vi "convertData.vi"(8 "error in (no error)":errorcluster, 10 "continuous":bool=TRUE, 11 "SpinCore in":refnum<class "SpinCore.lvclass">) -> (0 "error out":errorcluster, 2 "Instructions":T1(array[cluster]) {"Op Code" items=["Continue", "Stop", "Loop", "End Loop", "JSR", "RTS", "Branch", "Long Delay", "Wait"]; "Amp Register2" items=["0", "1", "2", "3"]; "Phase Register2" items=["0", "1", "2", "3", "4", "5", "6", "7", "8", "9", "10", "11", "12", "13", "14", "15"]; "Freq Register2" items=["0", "1", "2", "3", "4", "5", "6", "7", "8", "9", "10", "11", "12", "13", "14", "15"]; "Amp Register1" items=["0", "1", "2", "3"]; "Phase Register1" items=["0", "1", "2", "3", "4", "5", "6", "7", "8", "9", "10", "11", "12", "13", "14", "15"]; "Freq Register1" items=["0", "1", "2", "3", "4", "5", "6", "7", "8", "9", "10", "11", "12", "13", "14", "15"]; "Length" format="%.3p"}, 3 "SpinCore out":refnum<class "SpinCore.lvclass">)   [LabVIEW 2009, in "Hardware.lvlib" / "Channels.lvlib" / "SpinCore.lvclass"]
uses:
  SpinCore.lvclass
  SpinCore.lvclass/SpinCore.ctl
panel:
  # "0"
  # "1"
  # "2"
  # "3"
  # "4"
  # "5"
  # "6"
  # "7"
  # "8"
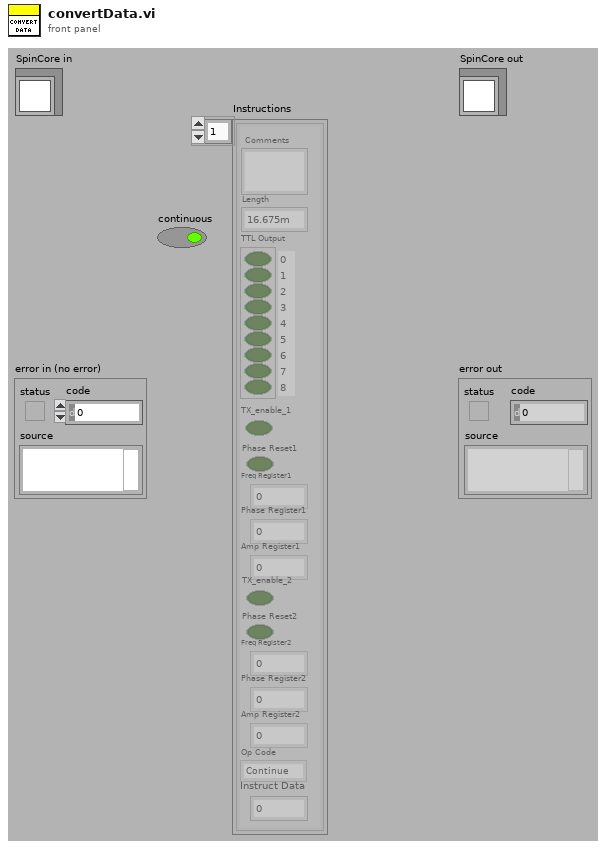
[diagram p1: front panel]
types:
  T1 = cluster{"Comments":string, "Length":dbl, "TTL Output":bool[], "TX_enable_1":bool, "Phase Reset1":bool, "Freq Register1":i32, "Phase Register1":i32, "Amp Register1":i32, "TX_enable_2":bool, "Phase Reset2":bool, "Freq Register2":i32, "Phase Register2":i32, "Amp Register2":i32, "Instruct Data":i32, "Op Code":i32}[]
  T2 = cluster{"Comments":string, "Length":dbl, "TTL Output":bool[], "TX_enable_0":bool, "Phase Reset0":bool, "Freq Register0":i32, "Phase Register0":i32, "Amp Register0":i32, "TX_enable_1":bool, "Phase Reset1":bool, "Freq Register1":i32, "Phase Register1":i32, "Amp Register1":i32, "Instruct Data":i32, "Op Code":i32}[]
  T3 = cluster{"Comments":string, "Length":dbl, "TTL Output":bool[], "TX_enable_1":bool, "Phase Reset1":bool, "Freq Register1":i32, "Phase Register1":i32, "Amp Register1":i32, "TX_enable_2":bool, "Phase Reset2":bool, "Freq Register2":i32, "Phase Register2":i32, "Amp Register2":i32, "Instruct Data":i32, "Op Code":i32}
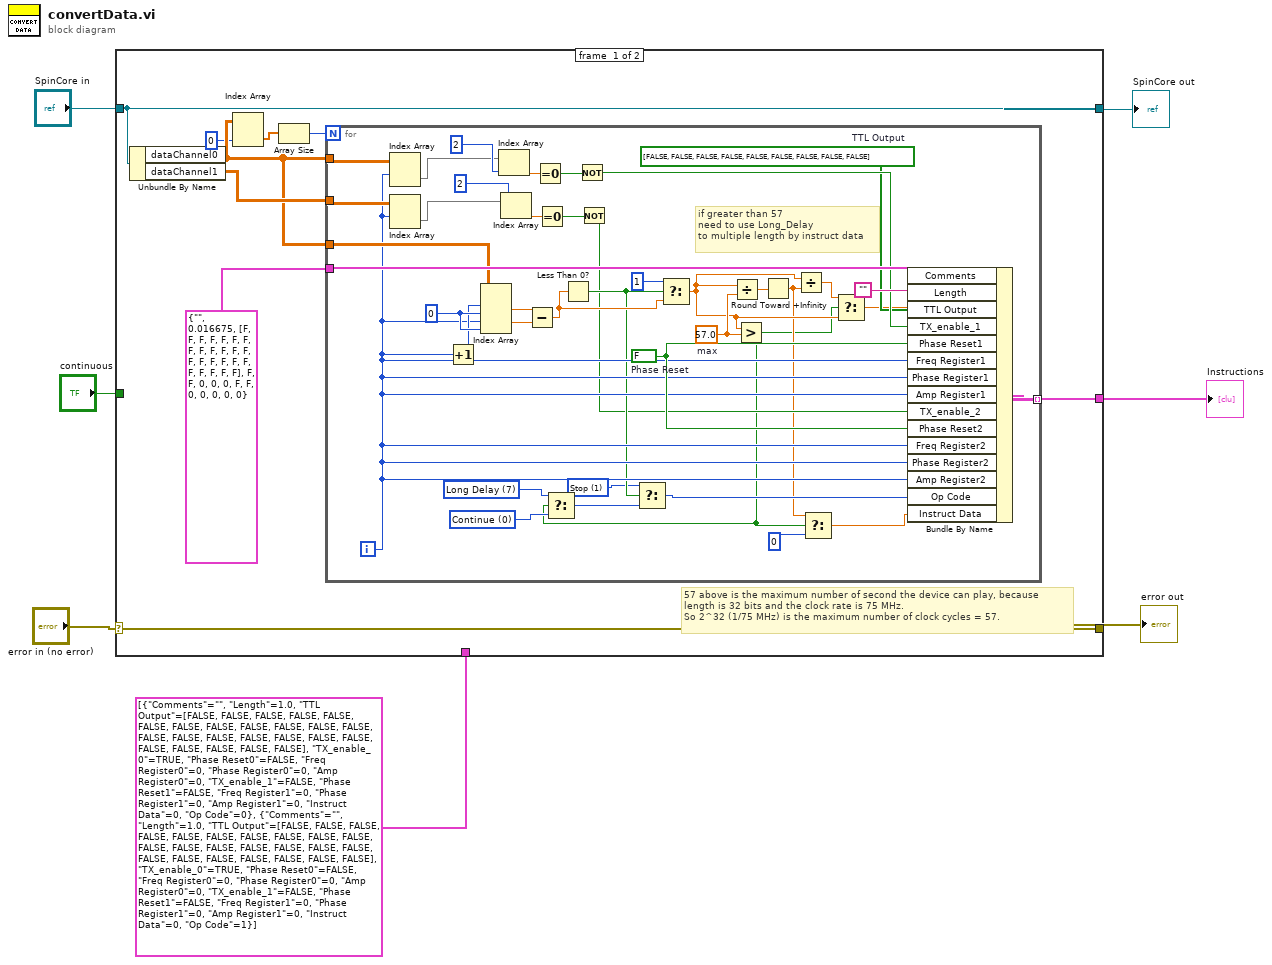
[diagram p0: block diagram]
diagram:
  n1 = case shown="No Error" "error in (no error)" {
    selector: "error in (no error)" -> [w16 w58]
    tunnel: [w16 w58] -> w6
    tunnel: [w15 w57] -> w4
    tunnel: "SpinCore in" -> [w15 w57]
    tunnel: [w8 _] -> w3
    tunnel: T2 [{"Comments"="", "Length"=1.0, "TTL Output"=[FALSE, FALSE, FALSE, FALSE, FALSE, FALSE, FALSE, FALSE, FALSE, FALSE, FALSE, FALSE, FALSE, FALSE, FALSE, FALSE, FALSE, FALSE, FALSE, FALSE, FALSE, FALSE, FALSE, FALSE], "TX_enable_0"=TRUE, "Phase Reset0"=FALSE, "Freq Register0"=0, "Phase Register0"=0, "Amp Register0"=0, "TX_enable_1"=FALSE, "Phase Reset1"=FALSE, "Freq Register1"=0, "Phase Register1"=0, "Amp Register1"=0, "Instruct Data"=0, "Op Code"=0}, {"Comments"="", "Length"=1.0, "TTL Output"=[FALSE, FALSE, FALSE, FALSE, FALSE, FALSE, FALSE, FALSE, FALSE, FALSE, FALSE, FALSE, FALSE, FALSE, FALSE, FALSE, FALSE, FALSE, FALSE, FALSE, FALSE, FALSE, FALSE, FALSE], "TX_enable_0"=TRUE, "Phase Reset0"=FALSE, "Freq Register0"=0, "Phase Register0"=0, "Amp Register0"=0, "TX_enable_1"=FALSE, "Phase Reset1"=FALSE, "Freq Register1"=0, "Phase Register1"=0, "Amp Register1"=0, "Instruct Data"=0, "Op Code"=1}] ("Instructions") -> [_ _]
    tunnel: "continuous" -> [_ _]
    frame #0 {
      # "57 above is the maximum number of second the device can play, because\nlength is 32 bits and the clock rate is 75 MHz.\nSo 2^32 (1/75 MHz) is the maximum number of clock cycles = 57."
      n2 = Unbundle By Name(w15) -> ("dataChannel0"=w13:dbl[][], "dataChannel1"=w14:dbl[][])
      n3 = Index Array(array=w13, index (col)=0) -> (element=w12:dbl[])  [unwired: 1 in]
      n4 = Array Size(array=w12) -> (size(s)=w10:i32)
      n5 = for {
        N: w10 -> [_]
        tunnel: w13 -> [w39]
        tunnel: w14 -> [w37]
        tunnel: T3 {"Comments"="", "Length"=0.016675, "TTL Output"=[FALSE, FALSE, FALSE, FALSE, FALSE, FALSE, FALSE, FALSE, FALSE, FALSE, FALSE, FALSE, FALSE, FALSE, FALSE, FALSE, FALSE, FALSE, FALSE, FALSE, FALSE, FALSE, FALSE, FALSE], "TX_enable_1"=FALSE, "Phase Reset1"=FALSE, "Freq Register1"=0, "Phase Register1"=0, "Amp Register1"=0, "TX_enable_2"=FALSE, "Phase Reset2"=FALSE, "Freq Register2"=0, "Phase Register2"=0, "Amp Register2"=0, "Instruct Data"=0, "Op Code"=0} ("DDS-II Instruction") -> [w50]
        tunnel: w13 -> [w48]
        tunnel: [w43] -> w8 mode=indexing
        i -> [w36]
        w23 = 57.0  # max
        w27 = 0 items=["Continue", "Stop", "Loop", "End Loop", "JSR", "RTS", "Branch", "Long Delay", "Wait"] ("Op Code")
        w33 = 1 items=["Continue", "Stop", "Loop", "End Loop", "JSR", "RTS", "Branch", "Long Delay", "Wait"] ("Op Code")
        w47 = 0
        w29 = bool[] [FALSE, FALSE, FALSE, FALSE, FALSE, FALSE, FALSE, FALSE, FALSE]  # TTL Output
        w49 = FALSE  # Phase Reset
        w26 = 7 items=["Continue", "Stop", "Loop", "End Loop", "JSR", "RTS", "Branch", "Long Delay", "Wait"] ("Op Code")
        # "if greater than 57\nneed to use Long_Delay\nto multiple length by instruct data"
        n6 = Index Array(array=w39, index (row)=w36) -> (element=w38:dbl[])  [unwired: 1 in]
        n7 = Index Array(array=w37, index (row)=w36) -> (element=w35:dbl[])  [unwired: 1 in]
        n8 = Increment(x=w36) -> (x+1=w46:i32)
        n9 = Index Array(array=w48, index (row) #1=w46, index (col) #1=w47, index (row) #2=w36, index (col) #2=w47) -> (element #1=w45:dbl, element #2=w44:dbl)
        n10 = Index Array(array=w38, index=2) -> (element=w55:dbl)
        n11 = Index Array(array=w35, index=2) -> (element=w52:dbl)
        n12 = Subtract(x=w45, y=w44) -> (x-y=w41:dbl)
        n13 = Equal To 0?(x=w55) -> (x = 0?=w54:bool)
        n14 = Equal To 0?(x=w52) -> (x = 0?=w51:bool)
        n15 = Less Than 0?(x=w41) -> (x < 0?=w34:bool)
        n16 = Not(x=w54) -> (.not. x?=w30:bool)
        n17 = Not(x=w51) -> (.not. x?=w31:bool)
        n18 = Select(t=1, s=w34, f=w41) -> (s? t:f=w20:dbl)
        n19 = Divide(x=w20, y=w23) -> (x/y=w22:dbl)
        n20 = Greater?(x=w20, y=w23) -> (0:w17:bool)
        n21 = Select(t=w26, s=w17, f=w27) -> (s? t:f=w28:i32)
        n22 = Select(t=w33, s=w34, f=w28) -> (s? t:f=w32:i32)
        n23 = Round Toward +Infinity(x=w22) -> (ceil(x): smallest int >= x=w18:dbl)
        n24 = Divide(x=w20, y=w18) -> (x/y=w21:dbl)
        n25 = Select(t=w18, s=w17, f=0) -> (s? t:f=w24:dbl)
        n26 = Select(t=w21, s=w17, f=w20) -> (s? t:f=w19:dbl)
        n27 = Bundle By Name(cluster=w50, "Comments"="", "Length"=w19, "TTL Output"=w29, "TX_enable_1"=w30, "Phase Reset1"=w49, "Freq Register1"=w36, "Phase Register1"=w36, "Amp Register1"=w36, "TX_enable_2"=w31, "Phase Reset2"=w49, "Freq Register2"=w36, "Phase Register2"=w36, "Amp Register2"=w36, "Op Code"=w32, "Instruct Data"=w24) -> (w43:T3)
      }
    }
    frame #1 {
    }
  }
  "error out" <- w6
  "SpinCore out" <- w4
  "Instructions" <- w3
